vi "Get_Time_Date.vi"() -> (0 "minute":i32, 1 "second":i32, 2 "fractional second":dbl, 3 "time string":string, 4 "hour":i32, 5 "DST":i32, 6 "day of year":i32, 7 "date string":string)   [LabVIEW 2020]
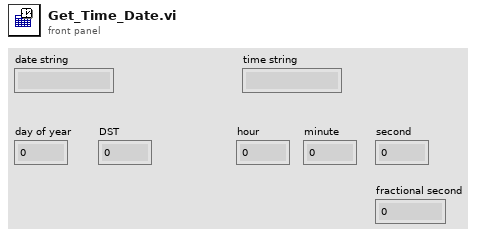
[diagram p1: front panel]
types:
  T1 = typedef "LVDateTimeRec.ctl" = cluster{"fractional second":dbl, "second":i32, "minute":i32, "hour":i32, "day of month":i32, "month":i32, "year":i32, "day of week":i32, "day of year":i32, "DST":i32}
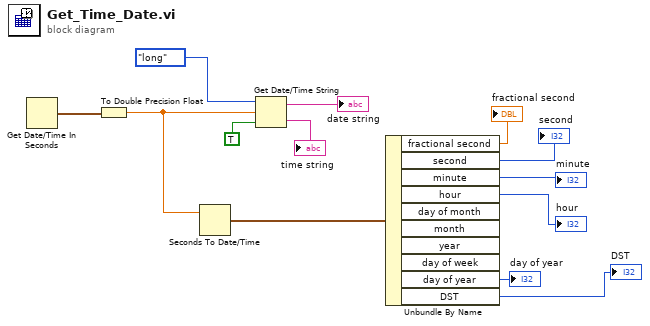
[diagram p0: block diagram]
diagram:
  n1 = Get Date/Time In Seconds() -> (seconds since 1Jan1904=w13:timestamp)
  n2 = To Double Precision Float(number=w13) -> (double precision float=w2:dbl)
  n3 = Seconds To Date/Time(time stamp (now)=w2) -> (date time rec=w8:T1)  [unwired: 1 in]
  n4 = Get Date/Time String(date format (0)=enum16{"short", "long", "abbreviated"}."long", seconds (now)=w2, want seconds? (F)=TRUE) -> (date string=→"date string":string, time string=→"time string":string)
  n5 = Unbundle By Name(w8) -> ("fractional second"=→"fractional second":dbl, "second"=→"second":i32, "minute"=→"minute":i32, "hour"=→"hour":i32, "day of year"=→"day of year":i32, "DST"=→"DST":i32)  [unwired: 4 out]
